vi "SendToAll.vi"(6 "Priority Message? (F)":bool, 8 "error in (no error)":errorcluster, 9 "Data":variant, 10 "Message":string, 11 "Message Queues in":T1) -> (0 "error out":errorcluster)   [LabVIEW 2017, in "Server.lvlib"]
doc: "Sends a Message to all Message-Queues except the MHL. This is used for broadcasting Initialize and Exit Messages (and maybe others that every loop needs)."
uses:
  Server.lvlib
  SubLibs/Message Queue/CommReferences.ctl
  SubLibs/Message Queue/MessageCluster.ctl
  SubLibs/Message Queue/EnqueueMessage(Single).vi
  SubLibs/Message Queue/Message Queue.lvlib
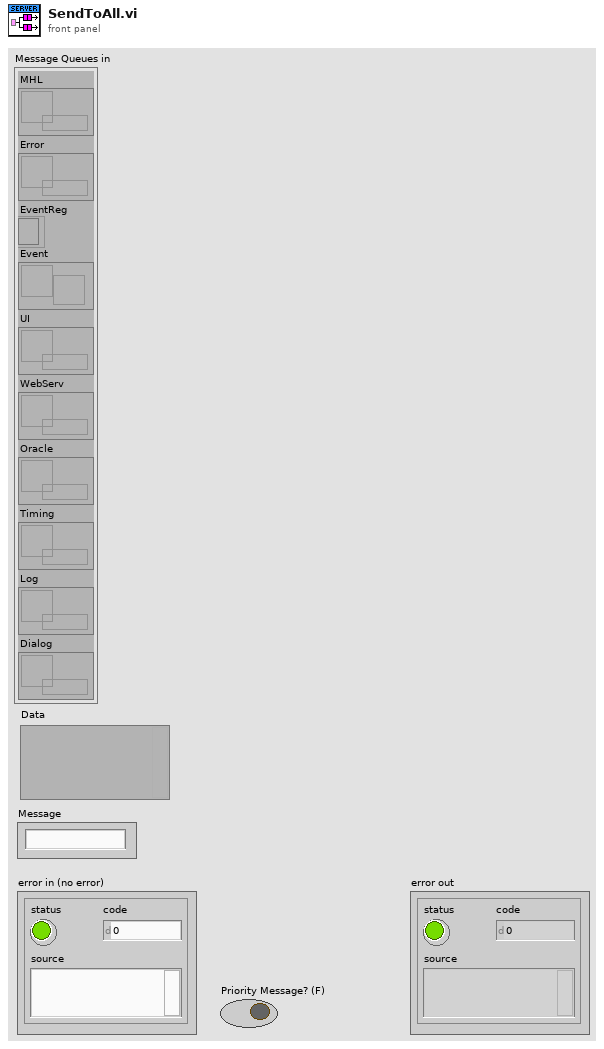
[diagram p1: front panel]
types:
  T1 = typedef "Server.lvlib/Message Queue.lvlib/CommReferences.ctl" = cluster{"MHL":refnum<queue>, "Error":refnum<queue>, "EventReg":refnum<event-registration>, "Event":refnum<user-event>, "UI":refnum<queue>, "WebServ":refnum<queue>, "Oracle":refnum<queue>, "Timing":refnum<queue>, "Log":refnum<queue>, "Dialog":refnum<queue>}
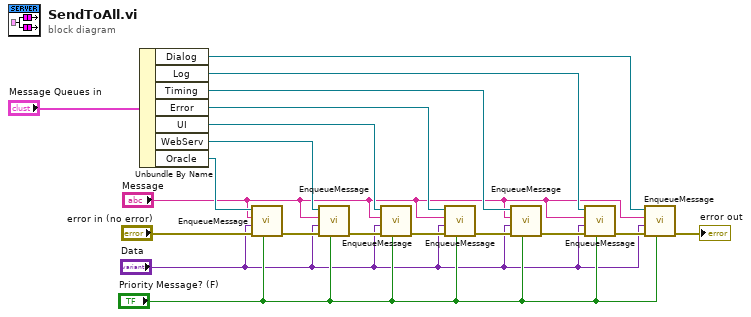
[diagram p0: block diagram]
diagram:
  n1 = Unbundle By Name("Message Queues in") -> ("Dialog"=w4:refnum<queue>, "Log"=w7:refnum<queue>, "Timing"=w19:refnum<queue>, "Error"=w17:refnum<queue>, "UI"=w16:refnum<queue>, "WebServ"=w15:refnum<queue>, "Oracle"=w14:refnum<queue>)
  n2 = call-poly "EnqueueMessage.vi"("Priority Message? (F)"="Priority Message? (F)", "error in (no error)"="error in (no error)", "Message Data"="Data", "Message"="Message", "Message Queue"=w14) -> ("error out"=w10:errorcluster)  [unwired: 5 in, 1 out]
  n3 = call-poly "EnqueueMessage.vi"("Priority Message? (F)"="Priority Message? (F)", "error in (no error)"=w10, "Message Data"="Data", "Message"="Message", "Message Queue"=w15) -> ("error out"=w11:errorcluster)  [unwired: 5 in, 1 out]
  n4 = call-poly "EnqueueMessage.vi"("Priority Message? (F)"="Priority Message? (F)", "error in (no error)"=w11, "Message Data"="Data", "Message"="Message", "Message Queue"=w16) -> ("error out"=w12:errorcluster)  [unwired: 5 in, 1 out]
  n5 = call-poly "EnqueueMessage.vi"("Priority Message? (F)"="Priority Message? (F)", "error in (no error)"=w12, "Message Data"="Data", "Message"="Message", "Message Queue"=w17) -> ("error out"=w18:errorcluster)  [unwired: 5 in, 1 out]
  n6 = call-poly "EnqueueMessage.vi"("Priority Message? (F)"="Priority Message? (F)", "error in (no error)"=w18, "Message Data"="Data", "Message"="Message", "Message Queue"=w19) -> ("error out"=w8:errorcluster)  [unwired: 5 in, 1 out]
  n7 = call-poly "EnqueueMessage.vi"("Priority Message? (F)"="Priority Message? (F)", "error in (no error)"=w8, "Message Data"="Data", "Message"="Message", "Message Queue"=w7) -> ("error out"=w6:errorcluster)  [unwired: 5 in, 1 out]
  n8 = call-poly "EnqueueMessage.vi"("Priority Message? (F)"="Priority Message? (F)", "error in (no error)"=w6, "Message Data"="Data", "Message"="Message", "Message Queue"=w4) -> ("error out"=→"error out":errorcluster)  [unwired: 5 in, 1 out]
